vi "0-360 deg Gyro Angle.vi"(1 "Raw Angle":dbl) -> (0 "0-360 deg Angle":dbl(knob) scale=0.0..360.0)   [LabVIEW 2015]
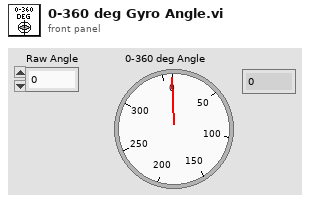
[diagram p1: front panel]
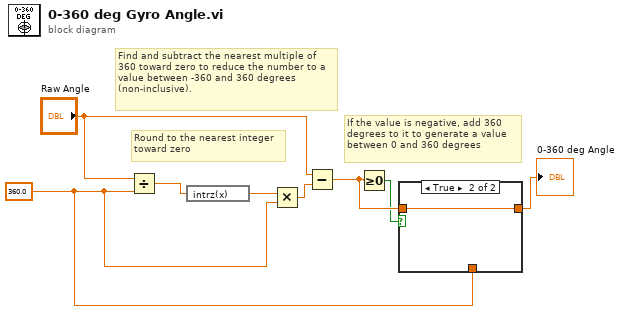
[diagram p0: block diagram]
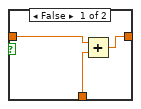
[diagram p2: hidden frame]
diagram:
  w5 = 360.0 ("y")
  # "If the value is negative, add 360 degrees to it to generate a value between 0 and 360 degrees"
  # "Find and subtract the nearest multiple of 360 toward zero to reduce the number to a value between -360 and 360 degrees (non-inclusive)."
  # "Round to the nearest integer toward zero"
  n1 = Divide(x="Raw Angle", y=w5) -> (x/y=w7:dbl)
  n2 = expression code="intrz(x)"(w7) -> (w6:dbl)
  n3 = Multiply(x=w6, y=w5) -> (x*y=w1:dbl)
  n4 = Subtract(x="Raw Angle", y=w1) -> (x-y=w4:dbl)
  n5 = Greater Or Equal To 0?(x=w4) -> (x >= 0?=w2:bool)
  n6 = case shown="True" w2 {
    tunnel: [w11 w12] -> w3
    tunnel: w4 -> [w9 w12]
    tunnel: w5 -> [w10 _]
    frame False {
      n7 = Add(x=w9, y=w10) -> (x+y=w11:dbl)
    }
    frame True {
    }
  }
  "0-360 deg Angle" <- w3
